vi "CS-4 Set Rates.vi"(2 "error in (no error)":errorcluster, 4 "sweep rates":T1={"rate 0"=0.5, "rate 1"=0.25, "rate 2"=0.1, "rate 3"=10.0} {"rate 3" min=0.0001 max=99.8 step=0.0001 format="%.4f"; "rate 2" min=0.0001 max=99.8 step=0.0001 format="%.4f"; "rate 1" min=0.0001 max=99.98 step=0.0001 format="%.4f"; "rate 0" min=0.0001 max=99.8 step=0.0001 format="%.4f"}, 5 "VISA session":refnum<visa-resource-name>) -> (0 "error out":errorcluster, 1 "dup VISA session":refnum<visa-resource-name>)   [LabVIEW 2016]
doc: "CS-4 Set Rates.vi sets the sweep rates for each sweep range and for fast mode. Rates 0-2 are the rates for each range and rate 3 is the rate used for fast mode"
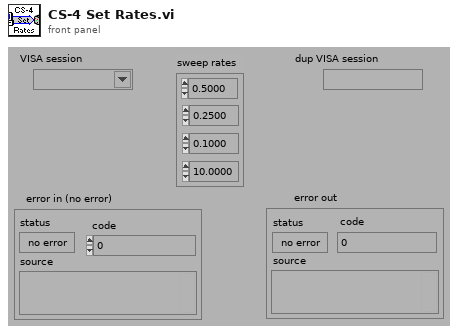
[diagram p1: front panel]
types:
  T1 = cluster{"rate 0":dbl, "rate 1":dbl, "rate 2":dbl, "rate 3":dbl}
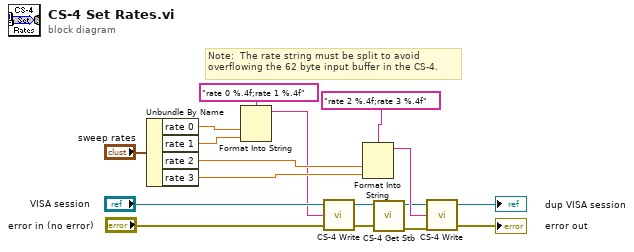
[diagram p0: block diagram]
diagram:
  # "Note:  The rate string must be split to avoid \noverflowing the 62 byte input buffer in the CS-4."
  n1 = Unbundle By Name("sweep rates") -> ("rate 0"=w9:dbl, "rate 1"=w8:dbl, "rate 2"=w7:dbl, "rate 3"=w6:dbl)
  n2 = Format Into String(format string="rate 0 %.4f;rate 1 %.4f", w9, w8) -> (resulting string=w5:string)  [unwired: 2 in, 1 out]
  n3 = call "CS-4 Write.vi"("error in (no error)"="error in (no error)", "write buffer (\"\")"=w5, "VISA session"="VISA session") -> ("error out"=w3:errorcluster, "dup VISA session"=w4:refnum<visa-resource-name>)  [unwired: 1 out]
  n4 = Format Into String(format string="rate 2 %.4f;rate 3 %.4f", w7, w6) -> (resulting string=w16:string)  [unwired: 2 in, 1 out]
  n5 = call "CS-4 Get Stb.vi"("error in (no error)"=w3, "VISA session"=w4) -> ("error out"=w1:errorcluster, "dup VISA session"=w2:refnum<visa-resource-name>)  [unwired: 2 in, 2 out]
  n6 = call "CS-4 Write.vi"("error in (no error)"=w1, "write buffer (\"\")"=w16, "VISA session"=w2) -> ("error out"=→"error out":errorcluster, "dup VISA session"=→"dup VISA session":refnum<visa-resource-name>)  [unwired: 1 out]
